vi "Gen_GetDeviceInformation.vi"(8 "error":errorcluster caption="错误输入（无错误）", 10 "Address":string) -> (0 "错误输出":errorcluster, 2 "Succeed":bool, 3 "Cards":T1[](array[typedef]), 4 "QXDAQ reference":refnum<k24>, 5 "QXSystem reference":refnum<k24>)   [LabVIEW 2016]
doc: "不连接Address接线端将从默认的配置文件中读取IP地址，\n连接Address接线端将使用输入的IP地址，并将该地址写入默认配置文件中。"
uses:
  DAQ-Config/Controls/PSCHN_Channel Para.ctl
  DAQ-Config/Controls/PSCHN_Card Para.ctl
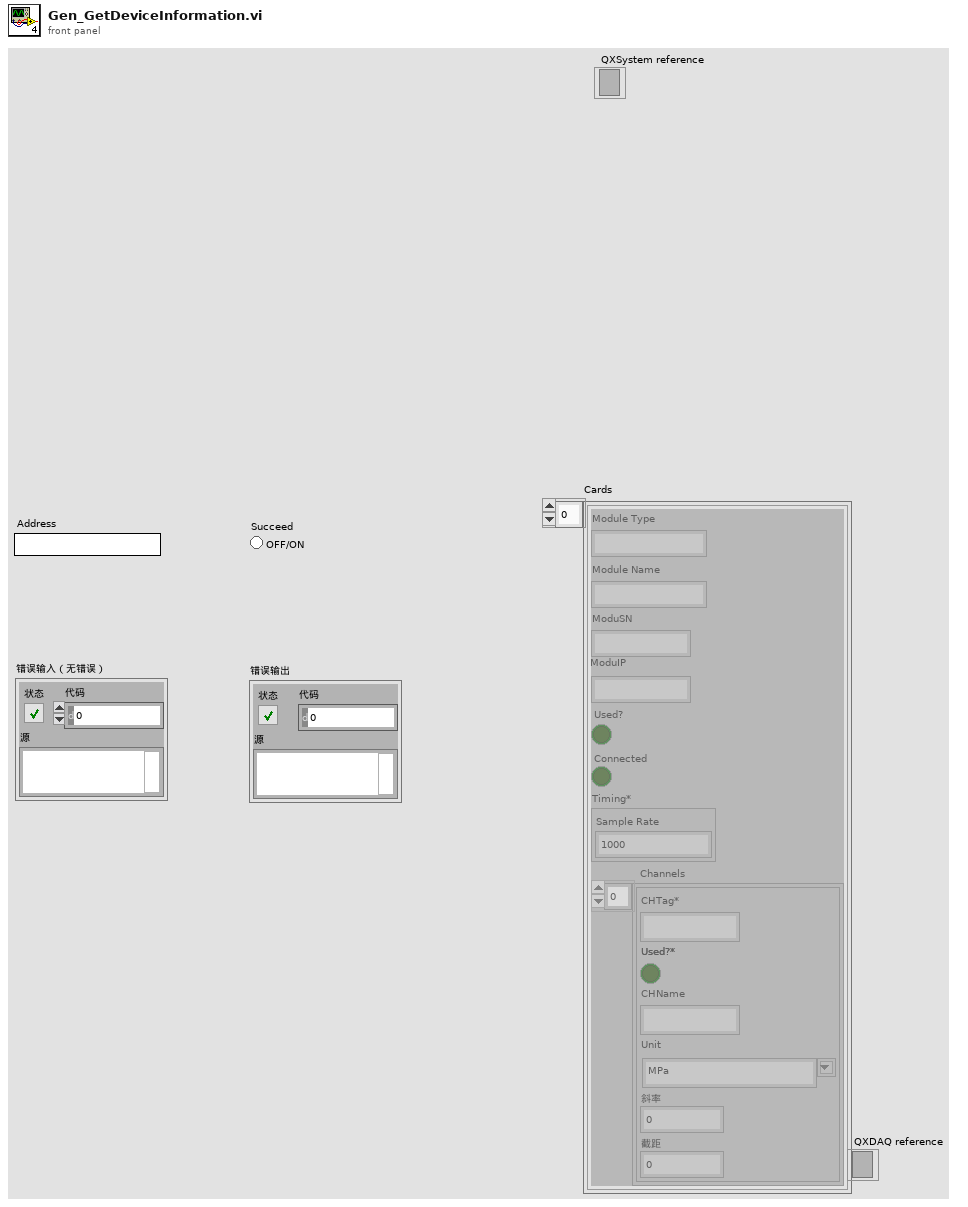
[diagram p1: front panel]
types:
  T1 = typedef "PSCHN_Card Para.ctl" = cluster{"Module Type":string, "Module Name":string, "ModuSN":string, "ModuIP":string, "Used?":bool, "Connected":bool, "Timing*":cluster{"Sample Rate":dbl}, "Channels":T2[]}
  T2 = typedef "PSCHN_Channel Para.ctl" = cluster{"CHTag*":string, "Used?*":bool, "CHName":string, "Unit":string, "斜率":dbl, "截距":dbl}
  T3 = typedef "QX_DeviceType.ctl" = cluster{"UUID":string, "Port":i32, "IP":string, "No Of Chans":i32, "Name":string}
  T4 = typedef "PSCHN_Channel Para.ctl" = cluster{"Channel Name*":string, "Used?*":bool, "Assign Name":string, "Save?*":bool, "Range":dbl, "Unit*":string, "Scale Result":string, "Channel Data*":variant, "斜率*":dbl, "截距*":dbl, "Electrical Zero":dbl, "Electrical Sensitivity":dbl, "Physical Zero*":dbl, "Physical Nominal":dbl, "Output rate*":dbl, "User Signal ID*":i32, "UUID*":string, "Connector number*":i32}
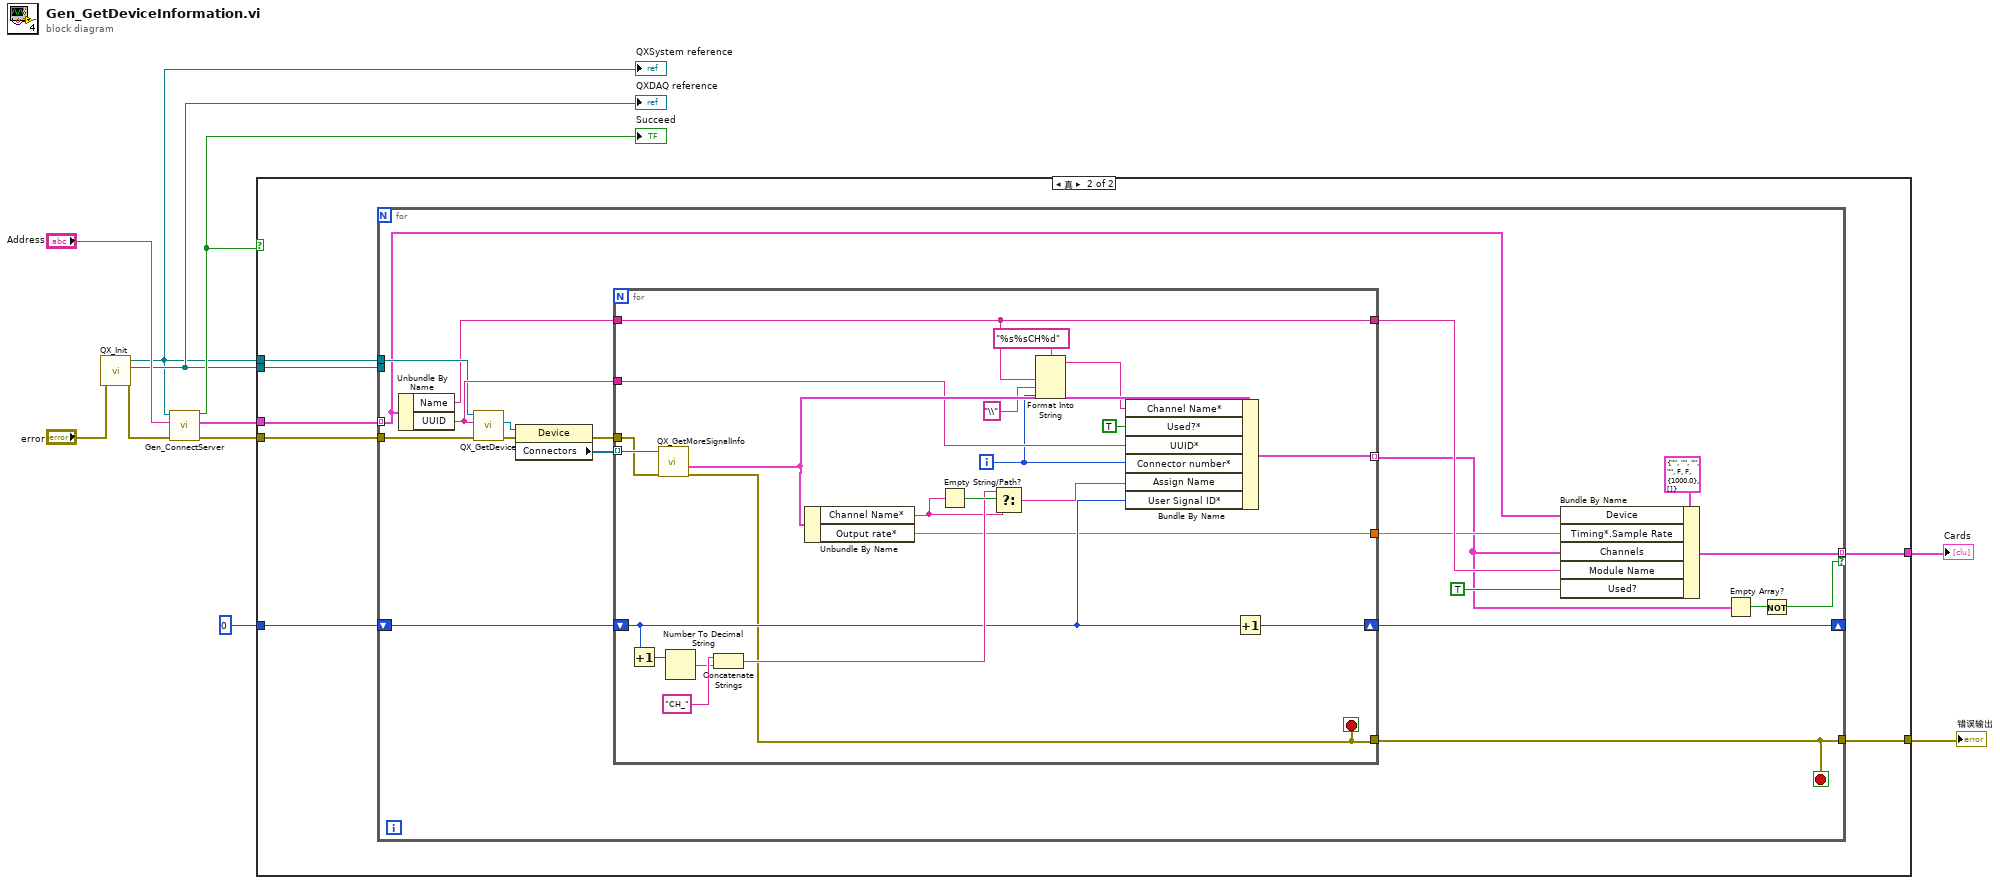
[diagram p0: block diagram]
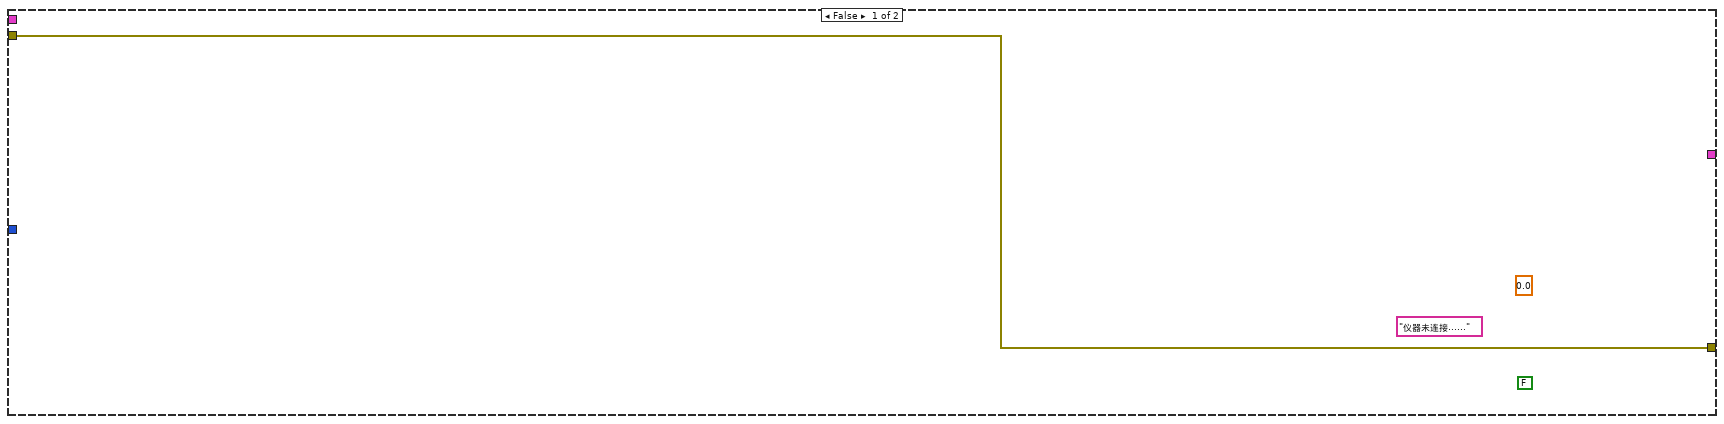
[diagram p2: hidden frame]
diagram:
  n1 = call <userlib>:"QX_Init.vi"("error in"="error") -> ("error out"=w7:errorcluster, "QXDAQ reference"=w5:refnum<k24>, "QXSystem reference"=w4:refnum<k24>)  [unwired: 8 in]
  "QXSystem reference" <- w4
  "QXDAQ reference" <- w5
  n2 = call "Gen_ConnectServer.vi"("QXSystem reference"=w4, "Address"="Address", "错误输入"=w7) -> ("Connect?"=w9:bool, "Devices"=w3:T3[], "错误输出"=w11:errorcluster)  [unwired: 5 in]
  "Succeed" <- w9
  n3 = case shown="真" w9 {
    tunnel: w11 -> [w12 w19]
    tunnel: [w12 w13] -> w8
    tunnel: w5 -> [_ w15]
    tunnel: w4 -> [_ w18]
    tunnel: w3 -> [_ w17]
    tunnel: 0 -> [_ w16]
    tunnel: [_ w14] -> w1
    frame False {
      (unwired) 0.0 ("HighSamplingFrequency")
      (unwired) FALSE
      (unwired) "仪器未连接......" ("Module Name")
    }
    frame True {
      n4 = for {
        tunnel: w17 -> [w24] mode=indexing
        tunnel: w19 -> [w33]
        tunnel: [w23] -> w13
        shift-right: [w34] -> _
        shift-left: w16 -> [w35]
        tunnel: w18 -> [w31]
        tunnel: w15 -> [_]
        tunnel: [w25] -> w14 mode=indexing if=w20
        stop <- w23 stop-if-true
        n5 = Unbundle By Name(w24) -> ("Name"=w30:string, "UUID"=w36:string)
        n6 = call <userlib>:"QX_GetDevice.vi"("error in"=w33, "UUID"=w36, "QXSystem reference"=w31) -> ("error out"=w39:errorcluster, "Device reference"=w38:refnum<k24>)  [unwired: 6 in, 1 out]
        n7 = property class="Device"(reference=w38, error in=w39) -> (error out=w32:errorcluster, "Connectors"=w37:refnum<k24>[])  [unwired: 1 out]
        n8 = for {
          tunnel: w37 -> [w57] mode=indexing
          tunnel: w36 -> [w51]
          shift-right: [w61] -> w34
          shift-left: w35 -> [w50]
          tunnel: w32 -> [w56]
          tunnel: [w40] -> w23
          tunnel: w30 -> [w43]
          tunnel: [w43] -> w27
          tunnel: [w48] -> w26
          tunnel: [w41] -> w22 mode=indexing
          i -> [w45]
          stop <- w40 stop-if-true
          n9 = Increment(x=w50) -> (x+1=w58:i32)
          n10 = call "QX_GetMoreSignalInfo.vi"("error in (no error)"=w56, "Connector Ref (Eingang)"=w57) -> ("Fehler (Ausgang)"=w40:errorcluster, "Channel out"=w52:T4)  [unwired: 8 in]
          n11 = Number To Decimal String(number=w58) -> (decimal integer string=w59:string)  [unwired: 1 in]
          n12 = Concatenate Strings("CH_" ("t"), w59) -> (w54:string)
          n13 = Unbundle By Name(w52) -> ("Channel Name*"=w53:string, "Output rate*"=w48:dbl)
          n14 = Empty String/Path?(string/path=w53) -> (empty?=w55:bool)
          n15 = Select(t=w54, s=w55, f=w53) -> (s? t:f=w49:string)
          n16 = Format Into String(format string="%s%sCH%d" ("格式字符串"), w43, "\\" ("输入 1"), w45) -> (resulting string=w42:string)  [unwired: 2 in, 1 out]
          n17 = Bundle By Name(cluster=w52, "Channel Name*"=w42, "Used?*"=TRUE, "UUID*"=w51, "Connector number*"=w45, "Assign Name"=w49, "User Signal ID*"=w50) -> (w41:T4)
          n18 = Increment(x=w50) -> (x+1=w61:i32)
        }
        n19 = Bundle By Name(cluster=T1 {"Module Type"="", "Module Name"="", "ModuSN"="", "ModuIP"="", "Used?"=FALSE, "Connected"=FALSE, "Timing*"={"Sample Rate"=1000.0}, "Channels"=[]} ("Card"), "Device"=w24, "Timing*.Sample Rate"=w26, "Channels"=w22, "Module Name"=w27, "Used?"=TRUE) -> (w25:T1)
        n20 = Empty Array?(array=w22) -> (empty?=w21:bool)
        n21 = Not(x=w21) -> (.not. x?=w20:bool)
      }
    }
  }
  "错误输出" <- w8
  "Cards" <- w1
